vi "Simulate Temperature Acquisition - Station 4.vi"() -> (3 "Temperature":dbl)   [LabVIEW 2019]
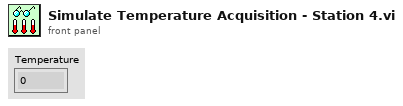
[diagram p1: front panel]
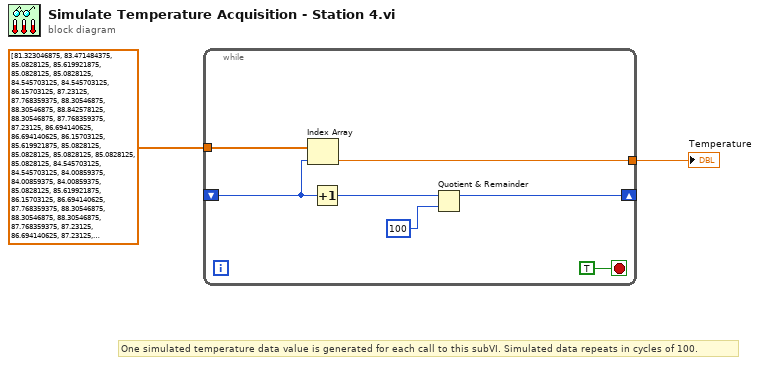
[diagram p0: block diagram]
diagram:
  # "One simulated temperature data value is generated for each call to this subVI. Simulated data repeats in cycles of 100."
  n1 = while {
    tunnel: dbl[] [81.323046875, 83.471484375, 85.0828125, 85.619921875, 85.0828125, 85.0828125, 84.545703125, 84.545703125, 86.15703125, 87.23125, 87.768359375, 88.30546875, 88.30546875, 88.842578125, 88.30546875, 87.768359375, 87.23125, 86.694140625, 86.694140625, 86.15703125, 85.619921875, 85.0828125, 85.0828125, 85.0828125, 85.0828125, 85.0828125, 84.545703125, 84.545703125, 84.00859375, 84.00859375, 84.00859375, 85.0828125, 85.619921875, 86.15703125, 86.694140625, 87.768359375, 88.30546875, 88.30546875, 88.30546875, 87.768359375, 87.23125, 86.694140625, 87.23125, 88.30546875, 88.842578125, 89.3796875, 88.842578125, 88.30546875, 88.30546875, 87.23125, 87.23125, 87.23125, 86.15703125, 86.15703125, 86.15703125, 85.619921875, 85.619921875, 86.694140625, 87.23125, 88.30546875, 88.30546875, 87.768359375, 87.23125, 86.694140625, 86.694140625, 86.15703125, 86.15703125, 85.619921875, 85.619921875, 85.0828125, 85.0828125, 84.545703125, 84.545703125, 84.00859375, 84.00859375, 84.00859375, 84.00859375, 84.00859375, 84.00859375, 84.00859375, 83.47124375, 81.86015625, 82.397265625, 83.47124375, 84.00859375, 83.471484375, 82.934375, 82.934375, 82.934375, 82.934375, 82.397265625, 82.397265625, 82.397265625, 82.397265625, 80.248828125, 80.248828125, 80.248828125, 80.248828125, 80.248828125, 80.248828125] ("array w/ subset deleted") -> [w8]
    tunnel: [w7] -> w2
    shift-right: [w5] -> _
    shift-left: _ -> [w3]
    stop <- TRUE stop-if-true
    n2 = Index Array(array=w8, index=w3) -> (element=w7:dbl)
    n3 = Increment(x=w3) -> (x+1=w4:i32)
    n4 = Quotient & Remainder(x=w4, y=100) -> (x-y*floor(x/y)=w5:i32)  [unwired: 1 out]
  }
  "Temperature" <- w2
